vi "cyfrowe - usun nieaktywne.vi"(6 "Array":bool[](array[boolean]), 7 "#cores (1)":i32=1, 8 "error in (no error)":errorcluster, 10 "Kanaly in":T1) -> (0 "error out":errorcluster, 2 "Kanaly out":T1)   [LabVIEW 2013]
doc: "Usuwa nieaktywne kanały cyfrowe\nAktywnym nadaje numerację kanału oraz właściwość aktywny"
uses:
  Kontrolki/Przetwarzanie/Kanaly.ctl
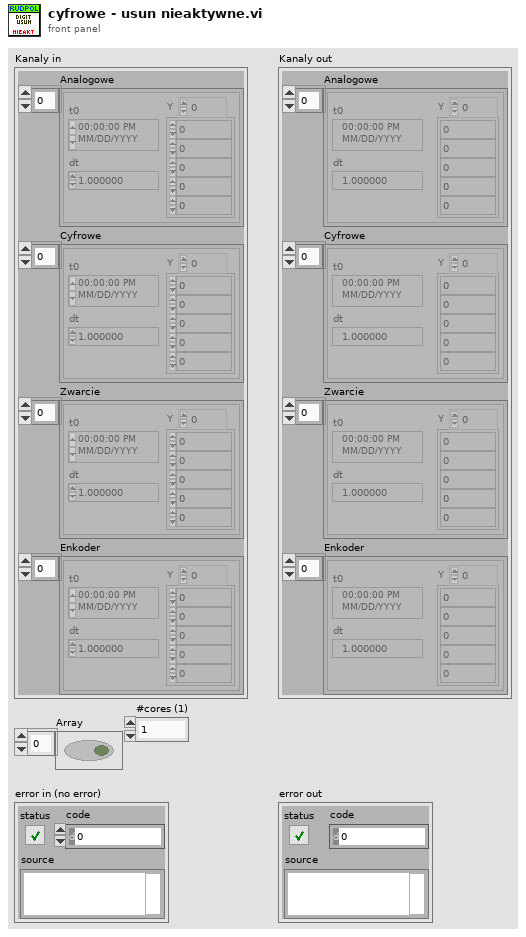
[diagram p1: front panel]
types:
  T1 = typedef "Kanaly.ctl" = cluster{"Analogowe":waveform(dbl)[], "Cyfrowe":waveform(dbl)[], "Zwarcie":waveform(dbl)[], "Enkoder":waveform(dbl)[]}
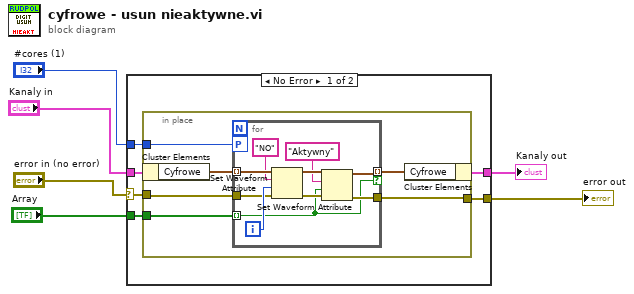
[diagram p0: block diagram]
diagram:
  n1 = case shown="No Error" "error in (no error)" {
    selector: "error in (no error)" -> [w8 w30]
    tunnel: [w12 w30] -> w6
    tunnel: "Array" -> [w11 _]
    tunnel: [w10 w29] -> w4
    tunnel: "Kanaly in" -> [w9 w29]
    tunnel: "#cores (1)" -> [w7 _]
    frame No Error {
      n2 = in-place {
        in-place-border: w11 -> [w16]
        in-place-border: w8 -> [w15]
        in-place-border: [w14] -> w12
        in-place-border: w7 -> [w13]
        n3 = in-place-cluster #1(w9) -> ("Cyfrowe"=w18:waveform(dbl)[])
        n4 = for {
          tunnel: w18 -> [w28] mode=indexing
          tunnel: [w21] -> w17 mode=indexing if=w19
          tunnel: w16 -> [w19] mode=indexing
          tunnel: w15 -> [w25]
          tunnel: [w20] -> w14
          workers-P: w13 -> [_]
          i -> [w27]
          n5 = Set Waveform Attribute(4:w25, 5:w27, 6:"NO", 7:w28) -> (0:w24:errorcluster, 3:w23:waveform(dbl))  [unwired: 1 out]
          n6 = Set Waveform Attribute(4:w24, 5:w19, 6:"Aktywny", 7:w23) -> (0:w20:errorcluster, 3:w21:waveform(dbl))  [unwired: 1 out]
        }
        n7 = in-place-cluster #1("Cyfrowe"=w17) -> (w10:T1)
      }
    }
    frame Error {
    }
  }
  "error out" <- w6
  "Kanaly out" <- w4
